vi "sub_deg4pid.vi"(9 "Heading":dbl, 10 "deg_gap":dbl, 11 "deg_target":dbl) -> (2 "heading for pid":dbl, 3 "deg-target for pid":dbl)   [LabVIEW 2019]
uses:
  Ctrl/state.ctl
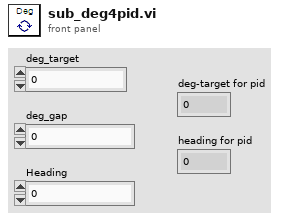
[diagram p1: front panel]
types:
  T1 = typedef "state.ctl" = enum16{"init", "Test circular track", "start point", "start heading adjust", "wait before start", "stop point check", "stop point start", "end point", "entering ending point", "move", "move heading adjust"}
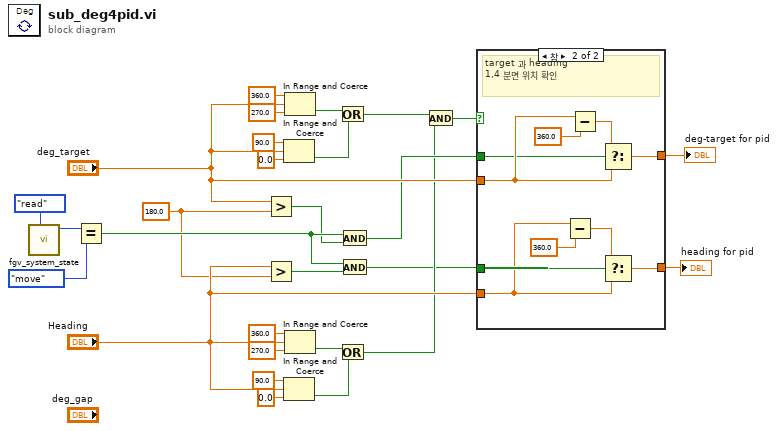
[diagram p0: block diagram]
diagram:
  w19 = 180.0 ("y")
  n1 = call "fgv_system_state.vi"("cmd"=enum16{"init", "read", "write"}."read") -> ("State out"=w24:T1)  [unwired: 9 in, 1 out]
  n2 = Equal?(x=w24, y=state."move") -> (x = y?=w27:bool)
  n3 = Greater?(x="deg_target", y=w19) -> (0:w4:bool)
  n4 = Greater?(x="Heading", y=w19) -> (0:w3:bool)
  n5 = In Range and Coerce(upper limit=90.0 ("상위 리미트"), x="deg_target", lower limit=0.0 ("하위 리미트")) -> (In Range?=w13:bool)  [unwired: 1 out]
  n6 = In Range and Coerce(upper limit=90.0 ("상위 리미트"), x="Heading", lower limit=0.0 ("하위 리미트")) -> (In Range?=w7:bool)  [unwired: 1 out]
  n7 = In Range and Coerce(upper limit=360.0 ("상위 리미트"), x="deg_target", lower limit=270.0 ("하위 리미트")) -> (In Range?=w14:bool)  [unwired: 1 out]
  n8 = In Range and Coerce(upper limit=360.0 ("상위 리미트"), x="Heading", lower limit=270.0 ("하위 리미트")) -> (In Range?=w8:bool)  [unwired: 1 out]
  n9 = Or(x=w14, y=w13) -> (x .or. y?=w5:bool)
  n10 = Or(x=w8, y=w7) -> (x .or. y?=w6:bool)
  n11 = And(x=w27, y=w4) -> (x .and. y?=w20:bool)
  n12 = And(x=w27, y=w3) -> (x .and. y?=w1:bool)
  n13 = And(x=w5, y=w6) -> (x .and. y?=w2:bool)
  n14 = case shown="참" w2 {
    tunnel: "deg_target" -> [w30 w36]
    tunnel: w20 -> [_ w35]
    tunnel: [w30 w34] -> w26
    tunnel: [w29 w33] -> w28
    tunnel: "Heading" -> [w29 w31]
    tunnel: w1 -> [_ w32]
    frame False {
    }
    frame True {
      # "target 과 heading \n1,4 분면 위치 확인"
      n15 = Subtract(x=w31, y=360.0) -> (x-y=w40:dbl)
      n16 = Subtract(x=w36, y=360.0) -> (x-y=w38:dbl)
      n17 = Select(t=w38, s=w35, f=w36) -> (s? t:f=w34:dbl)
      n18 = Select(t=w40, s=w32, f=w31) -> (s? t:f=w33:dbl)
    }
  }
  "heading for pid" <- w28
  "deg-target for pid" <- w26
